vi "Create and Register Sessions.vi"(8 "error in":errorcluster, 11 "sequence context":refnum<k7>) -> (0 "error out":errorcluster)   [LabVIEW 2020, in "NIDCPowerSourceDCVoltage.lvlib"]
uses:
  NIDCPowerSourceDCVoltage.lvlib
  <vilib>/MeasurementLink/MeasurementLink Session Management Client/RPC Messages/ni_measurementlink_PinMapContext.ctl
  <vilib>/MeasurementLink/MeasurementLink Session Management Client/MeasurementLink Session Management Client.lvlib
  <vilib>/MeasurementLink/MeasurementLink TestStand Integration/MeasurementLink TestStand Integration.lvlib
  <vilib>/MeasurementLink/MeasurementLink Session Management/Session Reservation/Session Reservation.lvclass
  <vilib>/MeasurementLink/MeasurementLink niDCPower/MeasurementLink niDCPower.lvlib
  <vilib>/MeasurementLink/MeasurementLink niDCPower/Create Sessions - NSess.vi
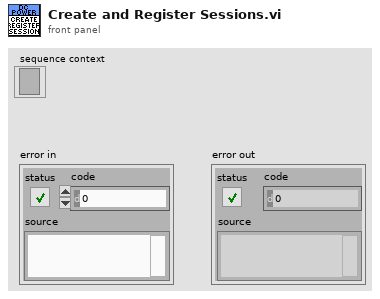
[diagram p1: front panel]
types:
  T1 = typedef "MeasurementLink Session Management Client.lvlib/ni_measurementlink_PinMapContext.ctl" = cluster{"pin_map_id":string, "sites":i32[]}
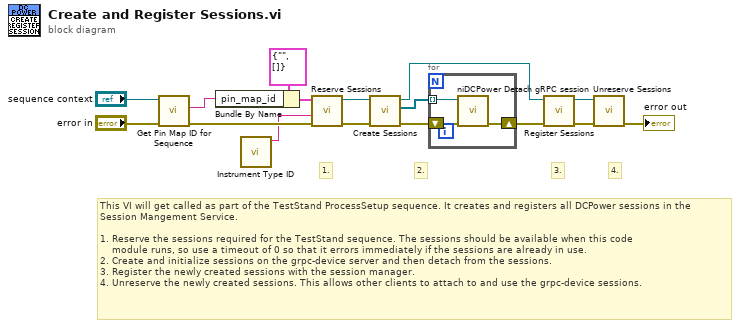
[diagram p0: block diagram]
diagram:
  # "4."
  # "3."
  # "2."
  # "1."
  # "This VI will get called as part of the TestStand ProcessSetup sequence. It creates and registers all DCPower sessions in the\nSession Mangement Service.\n\n1. Reserve the sessions required for the TestStand sequence. The sessions should be available when this code\n    module runs, so use a timeout of 0 so that it errors immediately if the sessions are already in use.  \n2. Create and initialize sessions on the grpc-device server and then detach from the sessions.\n3. Register the newly created sessions with the session manager.\n4. Unreserve the newly created sessions. This allows other clients to attach to and use the grpc-device sessions."
  n1 = call <vilib>:"Get Pin Map ID for Sequence.vi"("error in"="error in", "sequence context in"="sequence context") -> ("error out"=w14:errorcluster, "pin map id"=w12:string)  [unwired: 7 in, 1 out]
  n2 = Bundle By Name(cluster=T1 {"pin_map_id"="", "sites"=[]} ("pin map context"), "pin_map_id"=w12) -> (w11:T1)
  n3 = call <vilib>:"Instrument Type ID.vi"() -> ("instrument type id"=w1:string)  [unwired: 11 in]
  n4 = call <vilib>:"Reserve Sessions.vi"("error in"=w14, "instrument type id"=w1, "pin map context"=w11) -> ("error out"=w6:errorcluster, "session reservation out"=w5:refnum<class "Session Reservation.lvclass">)  [unwired: 7 in]
  n5 = call-poly <vilib>:"Create Sessions.vi"("error in"=w6, "session reservation in"=w5) -> ("error out"=w3:errorcluster, "sessions"=w2:refnum<k15>[], "session reservation out"=w4:refnum<class "Session Reservation.lvclass">)  [unwired: 6 in, 1 out]
  n6 = for {
    shift-right: [w18] -> w10
    shift-left: w3 -> [w19]
    tunnel: w2 -> [w17] mode=indexing
    n7 = call <instrlib>:"niDCPower Detach gRPC session.vi"("error in (no error)"=w19, "instrument handle"=w17) -> ("error out"=w18:errorcluster)  [unwired: 9 in]
  }
  n8 = call <vilib>:"Register Sessions.vi"("error in"=w10, "session reservation in"=w4) -> ("error out"=w8:errorcluster, "session reservation out"=w9:refnum<class "Session Reservation.lvclass">)  [unwired: 8 in]
  n9 = call <vilib>:"Unreserve Sessions.vi"("error in"=w8, "session reservation in"=w9) -> ("error out"=→"error out":errorcluster)  [unwired: 9 in]
